vi "_Autofill API CmbBox.vi"(0 "CmbBox":refnum<vi>, 1 "Current Module (\"\" to Generate an ID)":string, 5 "CSM Name":string, 7 "API Name":string, 9 "Force? (F)":bool, 11 "error in (no error)":errorcluster, 12 "Interface-Filter":refnum<vi>) -> (15 "error out":errorcluster)   [LabVIEW 2017, in "DebugConsole.lvlib"]
uses:
  DebugConsole.lvlib
  _csmHelper/API with lvcsm Support/CSM-Helper API with lvcsm Support.lvlib
  _csmHelper/CSM-Helper.lvclass
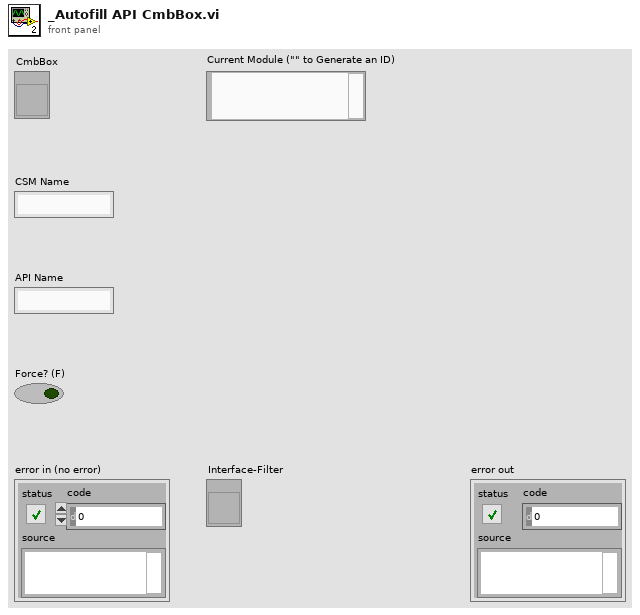
[diagram p1: front panel]
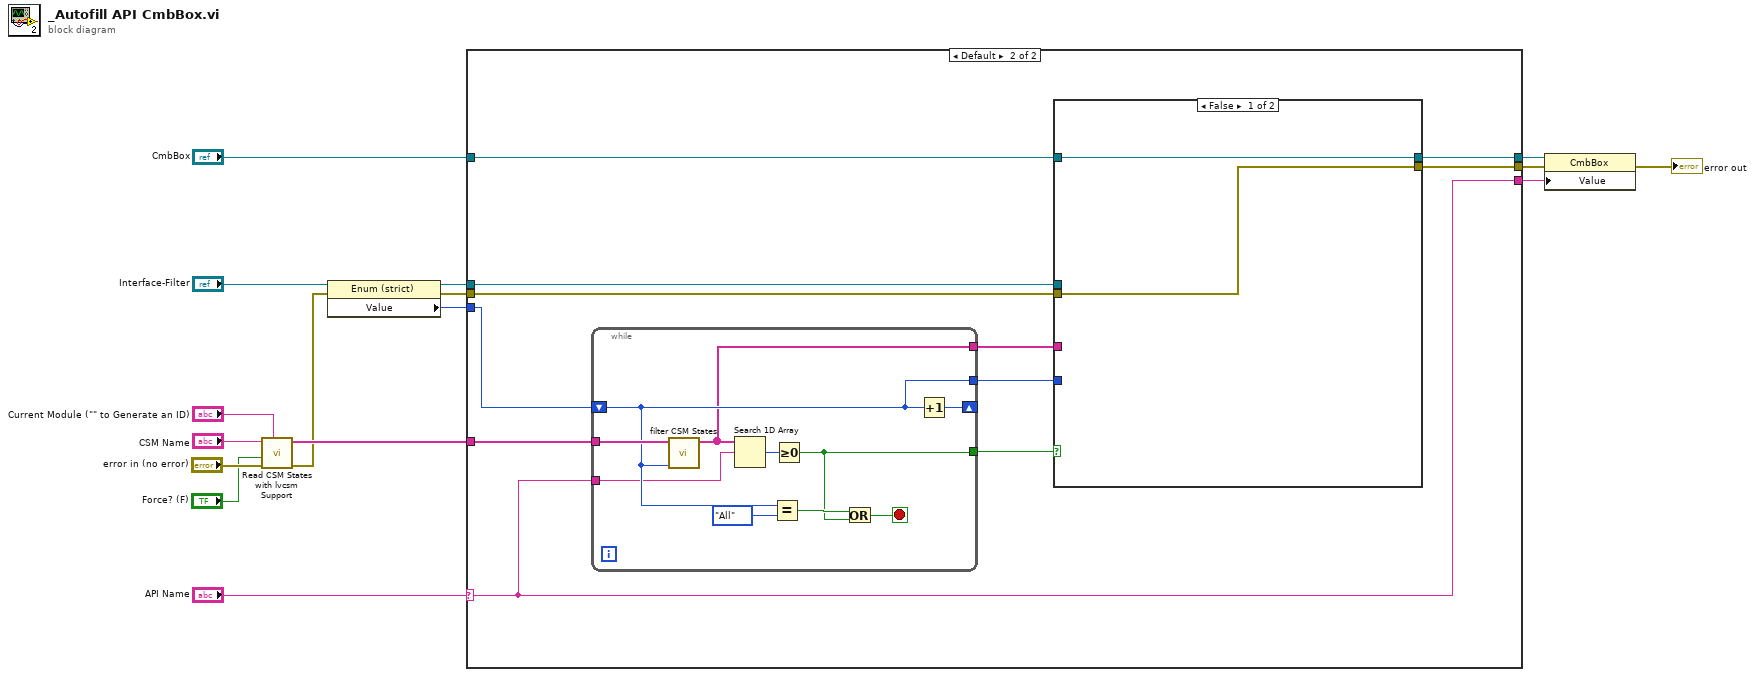
[diagram p0: block diagram]
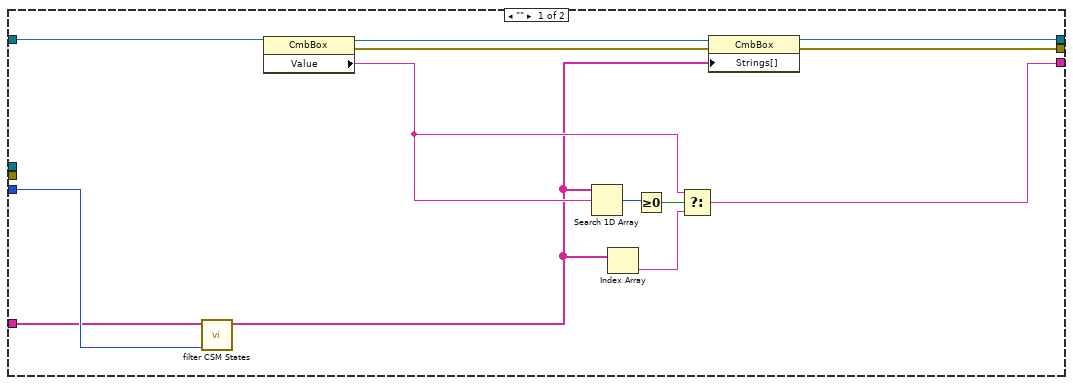
[diagram p2: hidden frame]
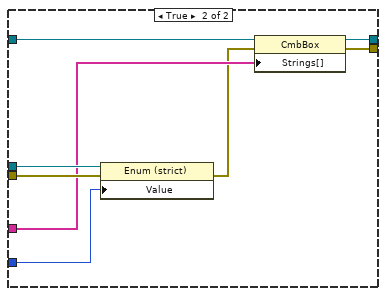
[diagram p3: hidden frame]
diagram:
  n1 = call "Read CSM States with lvcsm Support.vi"("Current Module (\"\" to Generate an ID)"="Current Module (\"\" to Generate an ID)", "error in (no error)"="error in (no error)", "Force? (F)"="Force? (F)", "CSM Name"="CSM Name") -> ("error out"=w7:errorcluster, "CSMAPI List"=w16:string[])  [unwired: 6 in]
  n2 = property on="Property Node" class="Enum (strict)"(reference="Interface-Filter", error in=w7) -> (reference out=w6:refnum<vi>, error out=w2:errorcluster, "Value"=w8:enum16{"API-Only", "UserDef States", "All"})
  n3 = case shown="Default" "API Name" {
    selector: "API Name" -> [_ w37]
    tunnel: w16 -> [w28 w40]
    tunnel: [w22 w37] -> w15
    tunnel: [w18 w32] -> w12
    tunnel: [w17 w31] -> w11
    tunnel: "CmbBox" -> [w27 w33]
    tunnel: w8 -> [w29 w35]
    tunnel: w6 -> [_ w39]
    tunnel: w2 -> [_ w38]
    frame "" {
      n4 = call "filter CSM States.vi"("Interface-Filter"=w29, "Array"=w28) -> ("filtered array"=w19:string[])  [unwired: 9 in]
      n5 = property on="Property Node" class="CmbBox"(reference=w27) -> (reference out=w20:refnum<vi>, error out=w21:errorcluster, "Value"=w24:string)  [unwired: 1 in]
      n6 = Search 1D Array(1D array=w19, element=w24) -> (index of element=w26:i32)  [unwired: 1 in]
      n7 = Index Array(array=w19) -> (element=w23:string)  [unwired: 1 in]
      n8 = Greater Or Equal To 0?(x=w26) -> (x >= 0?=w25:bool)
      n9 = Select(t=w24, s=w25, f=w23) -> (s? t:f=w22:string)
      n10 = property on="Property Node" class="CmbBox"(reference=w20, error in=w21, "Strings[]"=w19) -> (reference out=w18:refnum<vi>, error out=w17:errorcluster)
    }
    frame Default {
      n11 = while {
        tunnel: w40 -> [w59]
        shift-right: [w58] -> _
        shift-left: w35 -> [w55]
        tunnel: [w55] -> w36
        tunnel: [w53] -> w34
        tunnel: [w52] -> w30
        tunnel: w37 -> [w51]
        stop <- w57 stop-if-true
        n12 = call "filter CSM States.vi"("Interface-Filter"=w55, "Array"=w59) -> ("filtered array"=w53:string[])  [unwired: 9 in]
        n13 = Search 1D Array(1D array=w53, element=w51) -> (index of element=w60:i32)  [unwired: 1 in]
        n14 = Equal?(x=w55, y=enum16{"API-Only", "UserDef States", "All"}."All" ("Value")) -> (x = y?=w56:bool)
        n15 = Greater Or Equal To 0?(x=w60) -> (x >= 0?=w52:bool)
        n16 = Or(x=w56, y=w52) -> (x .or. y?=w57:bool)
        n17 = Increment(x=w55) -> (x+1=w58:enum16{"API-Only", "UserDef States", "All"})
      }
      n18 = case shown="False" w30 {
        tunnel: w39 -> [_ w50]
        tunnel: w38 -> [w41 w49]
        tunnel: w36 -> [_ w48]
        tunnel: w34 -> [_ w47]
        tunnel: w33 -> [w42 w46]
        tunnel: [w42 w45] -> w32
        tunnel: [w41 w43] -> w31
        frame False {
        }
        frame True {
          n19 = property on="Property Node" class="Enum (strict)"(reference=w50, error in=w49, "Value"=w48) -> (error out=w44:errorcluster)  [unwired: 1 out]
          n20 = property on="Property Node" class="CmbBox"(reference=w46, error in=w44, "Strings[]"=w47) -> (reference out=w45:refnum<vi>, error out=w43:errorcluster)
        }
      }
    }
  }
  n21 = property on="Property Node" class="CmbBox"(reference=w12, error in=w11, "Value"=w15) -> (error out=→"error out":errorcluster)  [unwired: 1 out]
